vi "Get User Config File Path.vi"(8 "Error In":errorcluster) -> (0 "Error Out":errorcluster, 3 "User Config refnum":T1)   [LabVIEW 2014]
uses:
  <vilib>/Utility/config.llb/Config Data RefNum.ctl
  <vilib>/Utility/config.llb/NI_LVConfig.lvlib
panel:
  out "file created?":bool
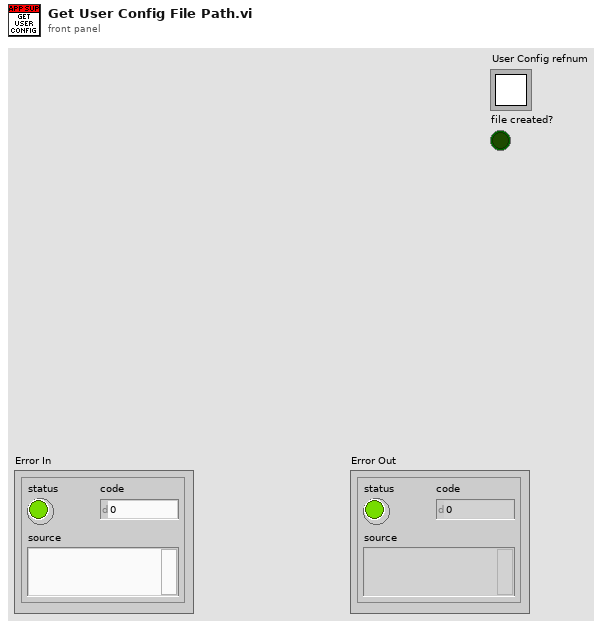
[diagram p1: front panel]
types:
  T1 = typedef "NI_LVConfig.lvlib/Config Data RefNum.ctl" = refnum<k1>
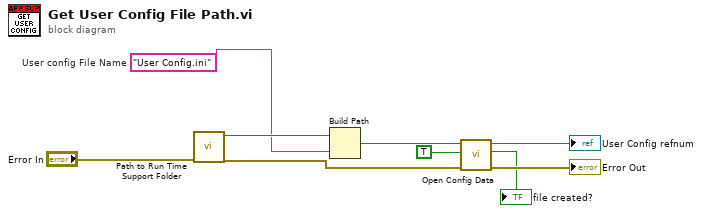
[diagram p0: block diagram]
diagram:
  w7 = "User Config.ini"  # User config File Name
  n1 = call "Path to Run Time Support Folder.vi"("Error In"="Error In") -> ("Error Out"=w3:errorcluster, "Path To Run Time Support Folder"=w9:path)  [unwired: 9 in]
  n2 = Build Path(base path=w9, name or relative path=w7) -> (appended path=w6:path)
  n3 = call <vilib>:"Open Config Data.vi"("error in (no error)"=w3, "create file if necessary (T)"=TRUE, "configuration file path"=w6) -> ("error out"=→"Error Out":errorcluster, "file created?"=→"file created?":bool, "refnum"=→"User Config refnum":T1)  [unwired: 6 in]
